vi "item.vi"(11 "Test.lvclass":refnum<class "Test.lvclass">) -> (3 "Test.lvclass 2":refnum<class "Test.lvclass">)   [LabVIEW 2010]
uses:
  Test.lvclass
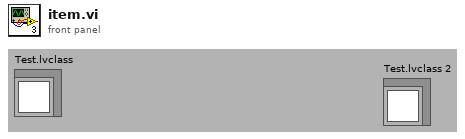
[diagram p1: front panel]
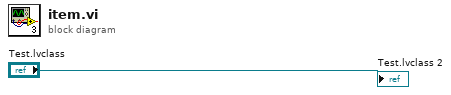
[diagram p0: block diagram]
diagram:
  "Test.lvclass 2" <- "Test.lvclass"
